vi "180122-uEye_Trigger_8bit-BM.vi"(6 "error in":errorcluster={"status"=TRUE, "code"=8, "source"="Create Folder in 170731-BM.vi<APPEND>\nC:\\Users\\FVMPE\\Desktop\\tmp\\BM"}, 8 "Phase":u16=1, 9 "Save Path":path=path "C:/Users/olfactory2P/Desktop/tmp/BM") -> (0 "error out":errorcluster={"status"=TRUE, "code"=50, "source"="LoadParameters.vi"} caption="error", 1 "DupFiles":bool)   [LabVIEW 2017]
doc: "SingleCapture_8bit nimmt ein Bilder von der Kamera auf und zeigt dieses an."
uses:
  <vilib>/vision/Image Controls.llb/IMAQ Image.ctl
  <vilib>/Analysis/_algsub.llb/Real Vector Norm.vi
  <vilib>/Analysis/Matrix/Numeric/Conversions/Array To Matrix - RA.vi
  Global_InitEndSync.vi
  <vilib>/Utility/file.llb/Write To Spreadsheet File (string).vi
  <vilib>/Analysis/Matrix/NI_Matrix.lvlib
  <vilib>/vision/NI_Vision_Development_Module.lvlib
  <vilib>/Analysis/NI_AALPro.lvlib
panel:
  in  "Settings":T1={"Objects"=1, "Threshold"=250, "Reject Border"=FALSE, "Fill Holes"=FALSE, "Min Object Size"=TRUE, "Min Size"=20, "Max Object Size"=FALSE, "Max Size"=100, "Show Search Area"=FALSE, "Show Center"=FALSE, "Show Bounding Box"=FALSE} {"Objects" items=["Bright Objects", "Dark Objects"]; "Threshold" min=1 max=999999999 step=1; "Max Size" min=1 max=999999999 step=1; "Min Size" min=1 max=999999999 step=1}
  in  "Threshold Limits":cluster{"Lower value":u8, "Upper value":u8}={"Lower value"=0, "Upper value"=66} {"Upper value" step=1 scale=0.0..255.0; "Lower value" step=1 scale=0.0..255.0}
  out "REC & Tracking State":string
  out "appended path":path
  in  "ROI to track":T2={"Left"=191, "Top"=183, "Right"=220, "Bottom"=212, "Rotation"=0.0} {"Rotation" format="%.2f"; "Left" scale=0.0..1024.0; "Right" scale=0.0..1024.0}
  out "Tracking":T3(plugin-control)
  in  "Shape Adapted Mean Shift ?":bool
  in  "Mean Shift Options in":T4={"Number of Histogram Bins"=10, "Blending Parameter (%)"=20.0, "Max Scale Change (%)"=0.0, "Max Rotation Change  (0-180 degree)"=70.0, "Max Shape Change (%)"=20.0, "Maximum Iterations"=15}
  out "Video":u8[][](graph)
  in  "Online Parameter Setting?":bool
  in  "Exposure":bool
  in  "Frame rate":u8(slide)=20 min=1 max=51 step=1 scale=1.0..50.17813236991319
  in  "Gamma":i32(slide) min=0 max=1000 step=100 scale=0.0..1000.0
  in  "Gamma":bool
  in  "Blacklevel Offset":i32(slide)=255 min=0 max=255 scale=0.0..255.0
  in  "Exposure Time":dbl(slide)=66.62091228070176 min=0.008982456140350877 max=66.62091228070176 step=0.05487719298245614 scale=0.008982456140350877..66.62091228070176 scale format="%#.3g"
  in  "Edge Filter Enable / Disable":bool
  in  "Edge Filter":i32(ring)=2 items=["High"=1, "Low"=2]
  in  "Blacklevel Compensation":bool
  in  "Hotpixel correction":bool
  in  "Master Gain":i32(slide)=100 min=0 max=100 scale=0.0..100.0
  in  "Autogain":bool
  in  "Load Parameter?":bool=TRUE
  in  "Parameter Path":path=path "C:/Users/olfactory2P/Documents/3mBM/CamParams/CamParam-180205-BM.ini"
  out "FPS":dbl=157.75358889414736
  in  "Camera ID":u32
  out "Get Trigger Mode":u16(ring)=4097 items=["Off"=0, "Hi-Low"=4097, "Low-Hi"=4098, "Software"=4104]
  in  "Trigger Mode":i32(ring)=4097 items=["IS_SET_TRIGGER_OFF"=0, "IS_SET_TRIGGER_HI_LO"=4097, "IS_SET_TRIGGER_LO_HI"=4098, "IS_SET_TRIGGER_SOFTWARE"=4104, "IS_GET_EXTERNALTRIGGER"=32768, "IS_GET_TRIGGER_STATUS"=32769]
  out "Height":i32=404
  out "Width":i32=404
  out "Bits/Pixel":i32=8
  in  "REC Stop":bool
  # "Setting"
  # "Image information"
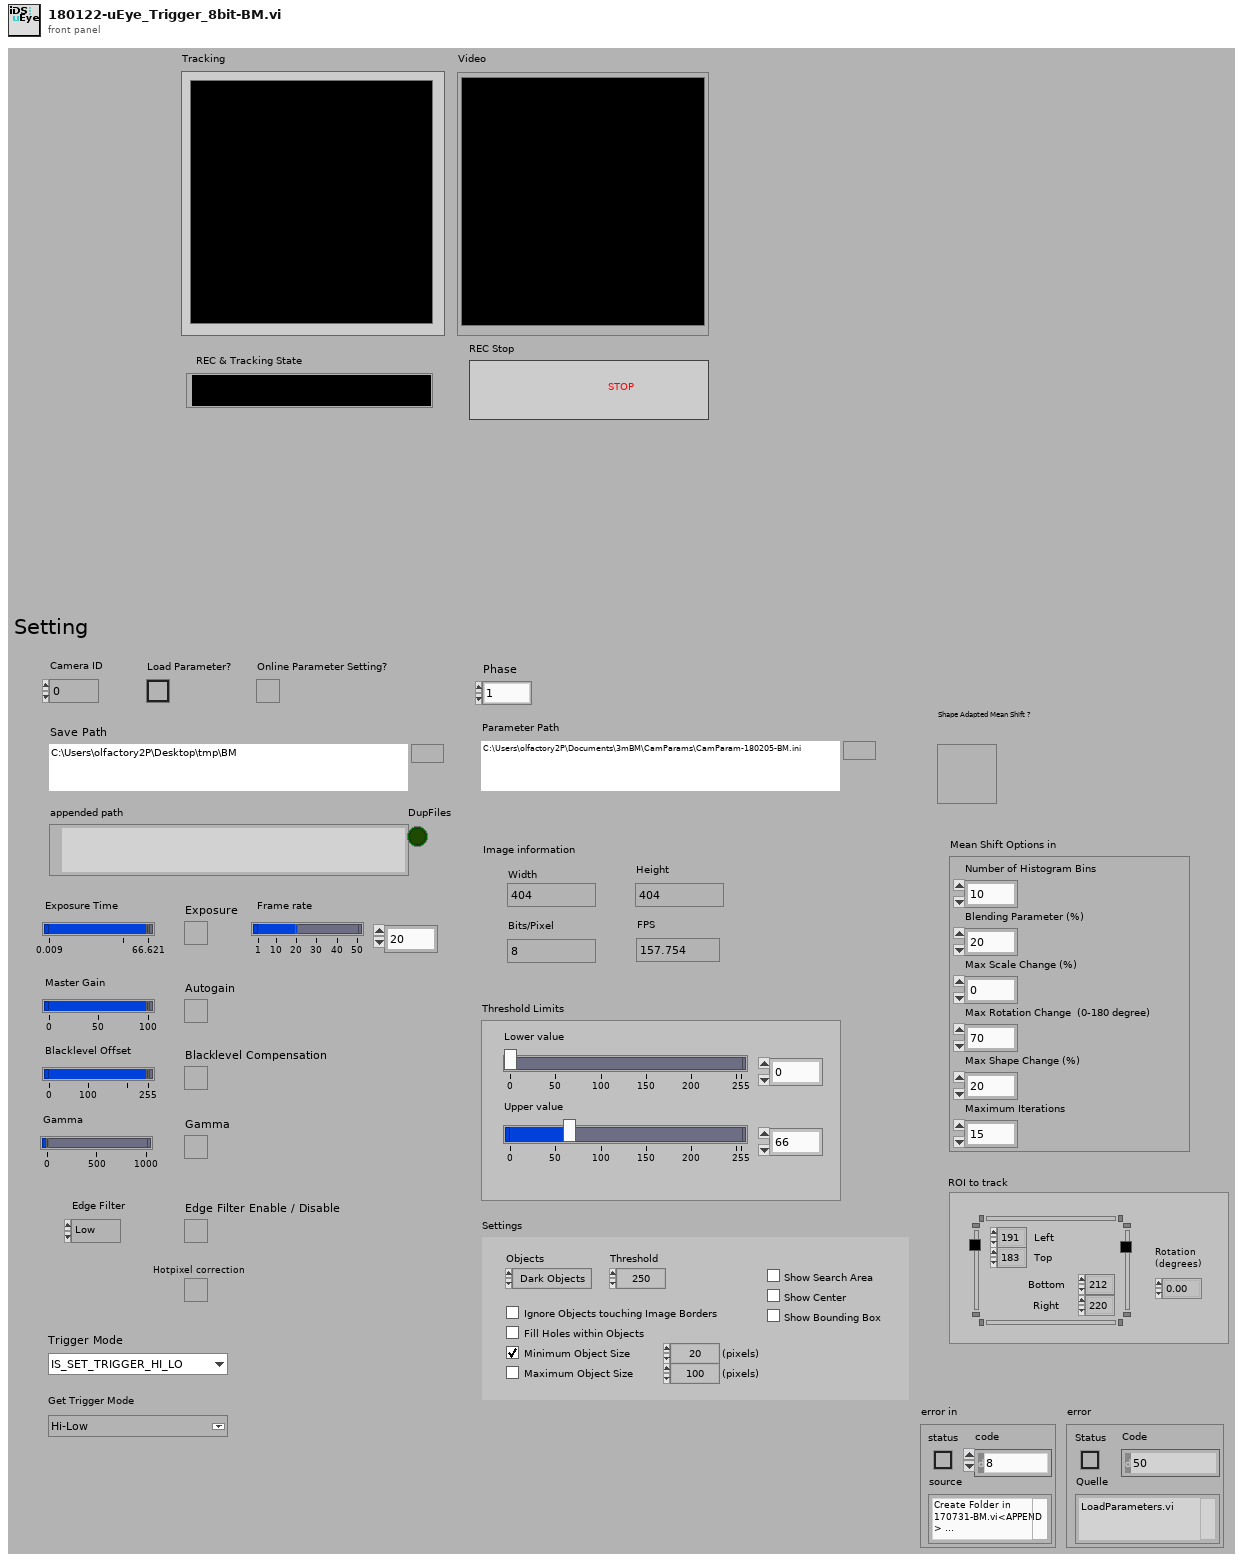
[diagram p1: front panel]
types:
  T1 = cluster{"Objects":u16, "Threshold":i32, "Reject Border":bool, "Fill Holes":bool, "Min Object Size":bool, "Min Size":i32, "Max Object Size":bool, "Max Size":i32, "Show Search Area":bool, "Show Center":bool, "Show Bounding Box":bool}
  T2 = typedef "IMAQ Rectangle" = cluster{"Left":i32, "Top":i32, "Right":i32, "Bottom":i32, "Rotation":dbl}
  T3 = typedef "IMAQ Image.ctl" = refnum<image>
  T4 = cluster{"Number of Histogram Bins":i32, "Blending Parameter (%)":dbl, "Max Scale Change (%)":dbl, "Max Rotation Change  (0-180 degree)":dbl, "Max Shape Change (%)":dbl, "Maximum Iterations":i32}
  T5 = typedef "IMAQ Object Tracking Session.ctl" = refnum<k20>
  T6 = cluster{"Number of Histogram Bins":i32, "Blending Parameter (%)":dbl, "Maximum Iterations":i32}
  T7 = typedef "IMAQ AVI2 Refnum.ctl" = refnum<k20>
  T8 = typedef "Image Type" = u32
  T9 = typedef "NI_Matrix.lvlib/RealMatrix.ctl" = dbl[][]
  T10 = cluster{"Left":i32, "Top":i32, "Right":i32, "Bottom":i32}
  T11 = typedef "ROI Descriptor" = cluster{"Global Rectangle":i32[], "Contours":cluster{"ID":enum32{"External", "Internal"}, "Type":u32, "Coordinates":i32[]}[]}
  T12 = cluster{"Label":string, "Score":i32, "Angle":dbl, "Location":cluster{"X":dbl, "Y":dbl}, "Bounding Box":cluster{"X":dbl, "Y":dbl}[], "Object Found?":bool}[]
  T13 = cluster{"Label":string, "Score":i32, "Angle":dbl, "Location":cluster{"X":dbl, "Y":dbl}, "Bounding Box":cluster{"X":dbl, "Y":dbl}[], "Object Found?":bool}
  T14 = cluster{"Object Center":cluster{"X":sgl, "Y":sgl}, "Bounding Box":cluster{"X Left":i32, "Y Top":i32, "X Right":i32, "Y Bottom":i32}, "Area":sgl, "Orientation":sgl, "Aspect Ratio":sgl, "Nb Holes":i32}[]
  T15 = cluster{"Object Center":cluster{"X":sgl, "Y":sgl}, "Bounding Box":cluster{"X Left":i32, "Y Top":i32, "X Right":i32, "Y Bottom":i32}, "Area":sgl, "Orientation":sgl, "Aspect Ratio":sgl, "Nb Holes":i32}
  T16 = cluster{"X Left":i32, "Y Top":i32, "X Right":i32, "Y Bottom":i32}
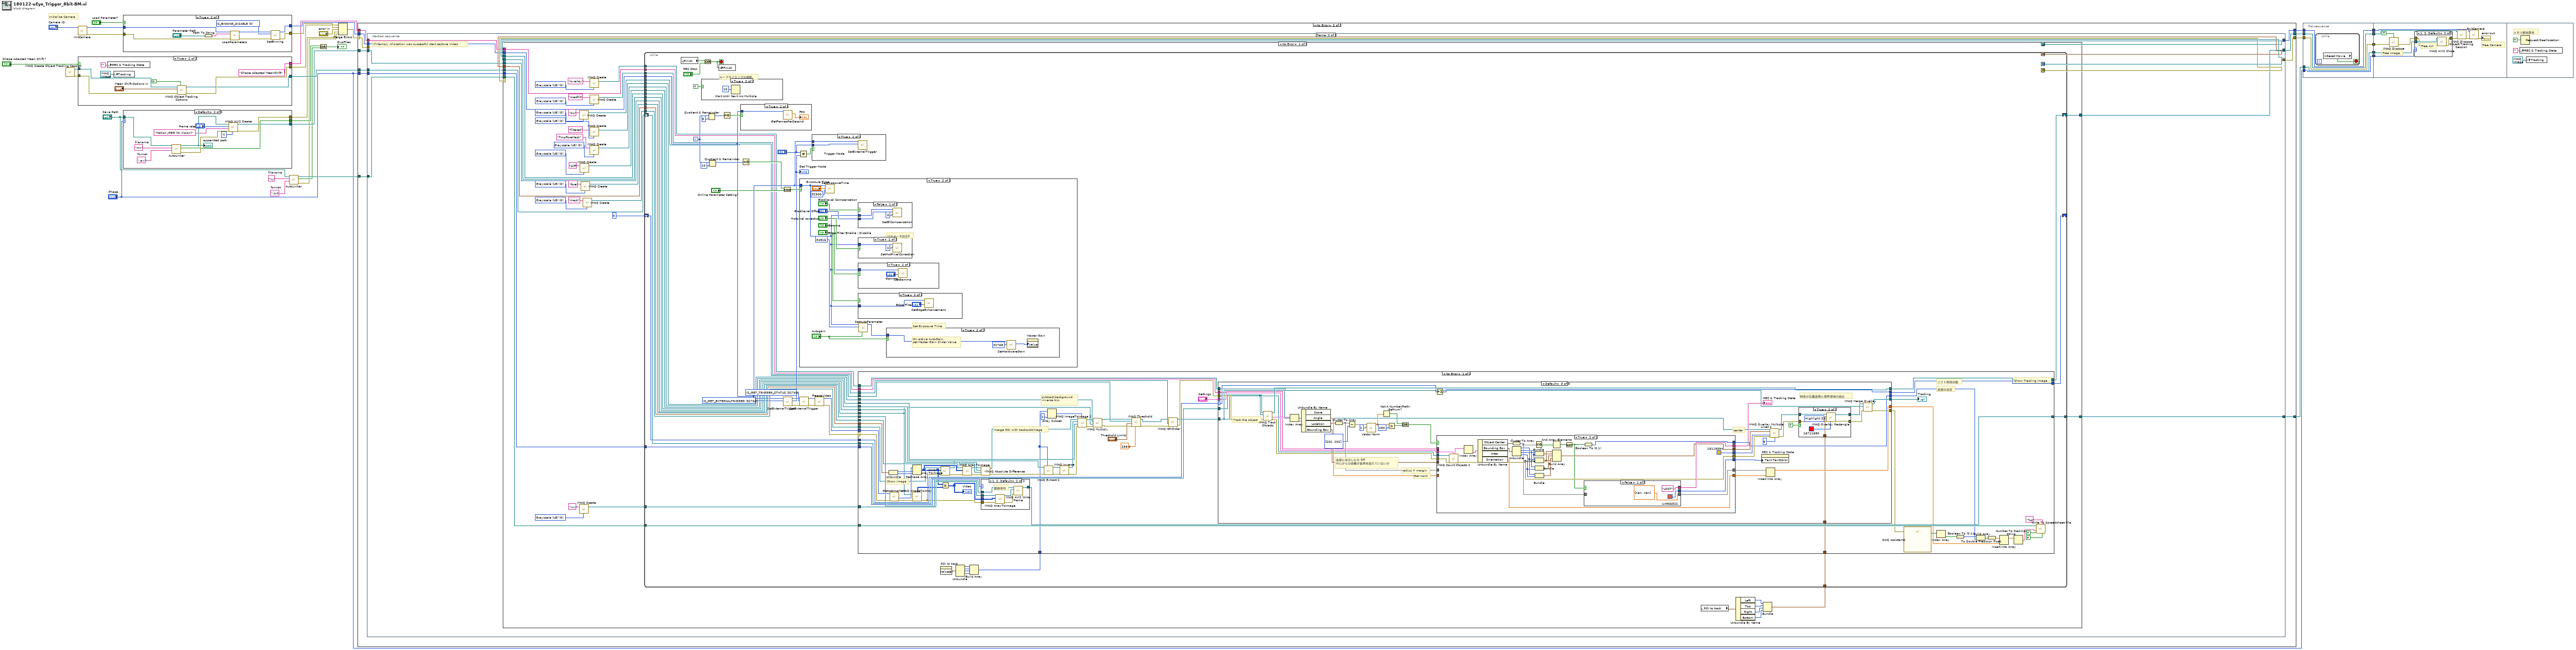
[diagram p0: block diagram]
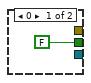
[diagram p2: hidden frame]
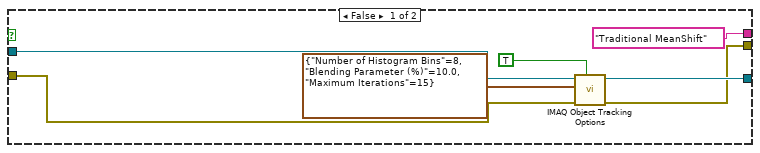
[diagram p3: hidden frame]
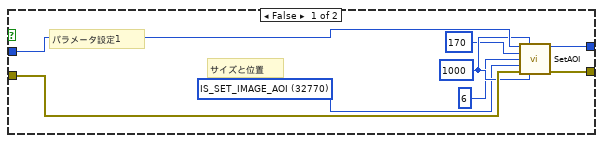
[diagram p5: hidden frame]
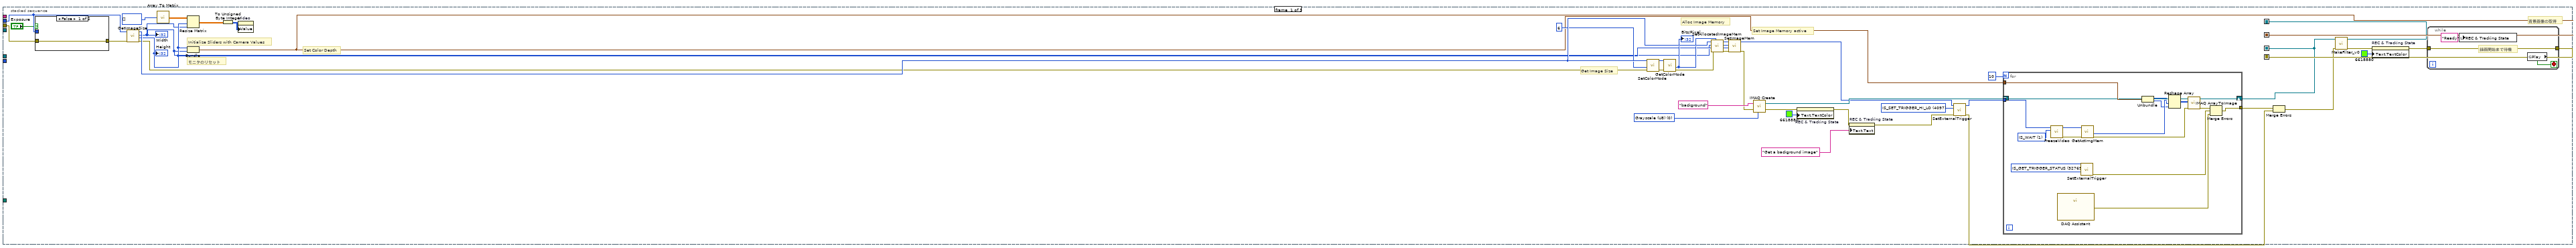
[diagram p7: hidden frame]
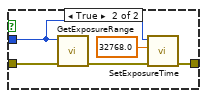
[diagram p8: hidden frame]
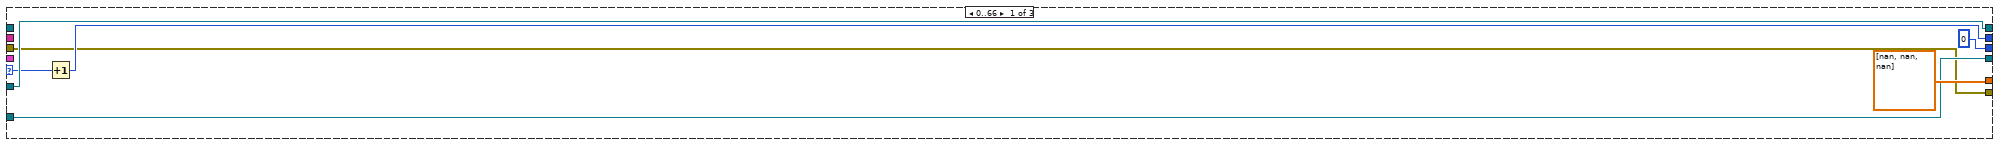
[diagram p10: hidden frame]
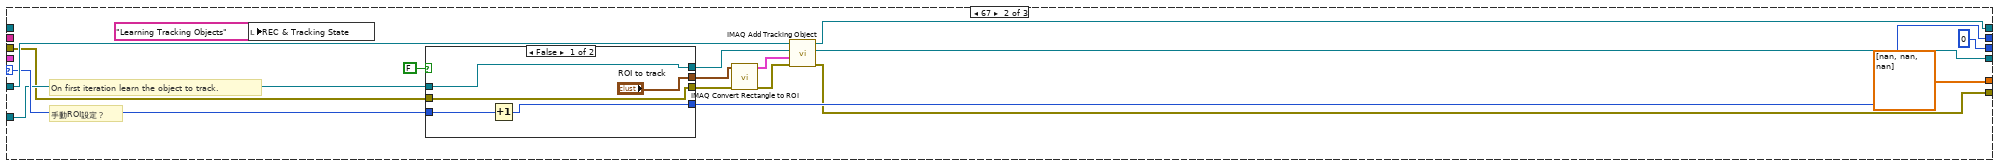
[diagram p11: hidden frame]
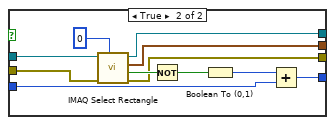
[diagram p12: hidden frame]
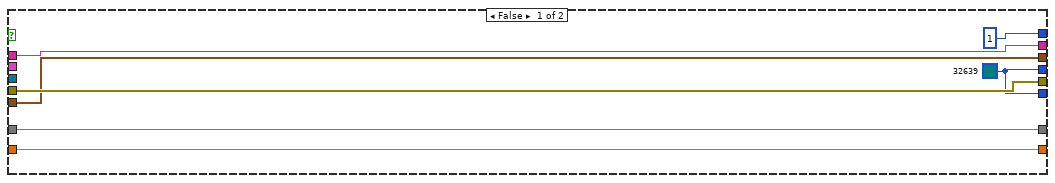
[diagram p14: hidden frame]
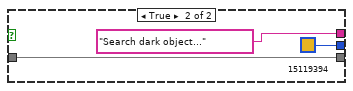
[diagram p15: hidden frame]
diagram:
  w14 = "xy"  # filename
  w13 = ".txt"  # format
  # "Initialize Camera"
  n1 = call "IMAQ Create Object Tracking Session"() -> ("error out"=w24:errorcluster, "Object Tracking Session"=w25:T5)  [unwired: 1 in, 9 out]
  n2 = call <instrlib>:"InitCamera.vi"("Camera ID"="Camera ID") -> ("error out"=w32:errorcluster, "Camera Handle Out"=w33:u32)  [unwired: 9 in]
  n3 = case shown="True" "Shape Adapted Mean Shift ?" {
    tunnel: w25 -> [w38 w50]
    tunnel: w24 -> [w37 w49]
    tunnel: [w39 w48] -> w21
    tunnel: [w40 w47] -> w20
    tunnel: ["Traditional MeanShift" "Shape Adapted MeanShift"] -> w7
    frame False {
      n4 = call-poly "IMAQ Object Tracking Options"("Get/Set (Get)"=TRUE, "error in (no error)"=w37, "Mean Shift Options in"=T6 {"Number of Histogram Bins"=8, "Blending Parameter (%)"=10.0, "Maximum Iterations"=15}, "Object Tracking Session In"=w38) -> ("error out"=w39:errorcluster, "Object Tracking Session Out"=w40:T5)  [unwired: 5 in, 1 out]
    }
    frame True {
      n5 = local write "REC & Tracking State"("") -> ()
      n6 = local write "Tracking"(T3 refnum ("Tracking")) -> ()
      n7 = call-poly "IMAQ Object Tracking Options"("Get/Set (Get)"=TRUE, "error in (no error)"=w49, "Shape Adapted Options in"="Mean Shift Options in", "Object Tracking Session In"=w50) -> ("error out"=w48:errorcluster, "Object Tracking Session Out"=w47:T5)  [unwired: 5 in, 1 out]
    }
  }
  n8 = case shown="True" "Load Parameter?" {
    tunnel: w33 -> [w58 w67]
    tunnel: [w51 w61] -> w27
    tunnel: w32 -> [w57 w66]
    tunnel: [w52 w60] -> w28
    frame False {
      w53 = 32770 items=["IS_SET_IMAGE_AOI"=32770, "IS_GET_IMAGE_AOI"=32771] ("Mode")
      w56 = 1000
      # "サイズと位置"
      # "パラメータ設定1"
      n9 = call <instrlib>:"SetAOI.vi"("Camera Handle In"=w58, "Width In"=w56, "XPos In"=170, "YPos In"=6, "Mode"=w53, "error in"=w57, "Height In"=w56) -> ("Camera Handle Out"=w51:u32, "error out"=w52:errorcluster)  [unwired: 3 in, 4 out]
    }
    frame True {
      w59 = 0 items=["IS_BINNING_DISABLE"=0, "IS_BINNING_2X_VERTICAL"=1, "IS_BINNING_2X_HORIZONTAL"=2, "IS_BINNING_4X_VERTICAL"=4, "IS_BINNING_4X_HORIZONTAL"=8, "IS_GET_BINNING"=32768, "IS_GET_SUPPORTED_BINNING"=32769] ("Mode")
      n10 = Path To String(path="Parameter Path") -> (string=w62:string)
      n11 = call <instrlib>:"LoadParameters.vi"("Camera Handle In"=w67, "Filename"=w62, "error in"=w66) -> ("Camera Handle Out"=w65:u32, "error out"=w64:errorcluster)  [unwired: 11 in]
      n12 = call <instrlib>:"SetBinning.vi"("error in"=w64, "Mode"=w59, "Camera Handle In"=w65) -> ("error out"=w60:errorcluster, "Camera Handle Out"=w61:u32)  [unwired: 6 in, 1 out]
    }
  }
  n13 = case shown="Default" "Phase" {
    tunnel: [_ w79] -> w19
    tunnel: "Save Path" -> [_ w77]
    tunnel: [_ w72] -> w15
    tunnel: [FALSE w71] -> w9
    frame 0 {
    }
    frame Default {
      w75 = "mv"  # filename
      w76 = ".avi"  # format
      n14 = call "AutoLinker.vi"("format"=w76, "filename"=w75, "Save Path"=w77) -> ("error out"=w73:errorcluster, "DupFiles"=w71:bool, "appended path"=w74:path)  [unwired: 6 in]
      "appended path" <- w74
      n15 = call "IMAQ AVI2 Create"("Quality"=-1, "error in (no error)"=w73, "Codec"="Motion JPEG (NI Vision)", "Frames Per Second"="Frame rate", "AVI Path"=w74) -> ("error out"=w72:errorcluster, "AVI Refnum"=w79:T7)  [unwired: 5 in]
    }
  }
  n16 = call "AutoLinker.vi"("format"=w13, "filename"=w14, "Save Path"="Save Path") -> ("error out"=w11:errorcluster, "DupFiles"=w10:bool, "appended path"=w16:path)  [unwired: 6 in]
  n17 = Or(x=w9, y=w10) -> (x .or. y?=→"DupFiles":bool)
  n18 = Merge Errors(w28, w21, "error in", w15, w11) -> (w30:errorcluster)
  n19 = case shown="No Error" w30 {
    selector: w30 -> [w80 w89]
    tunnel: [w81 w92] -> w29
    tunnel: w27 -> [w81 w91]
    tunnel: [w80 w90] -> w6
    tunnel: [_ w88] -> w26
    tunnel: w19 -> [_ w87]
    tunnel: w20 -> [_ w86]
    tunnel: "Phase" -> [_ w85]
    tunnel: [_ w84] -> w18
    tunnel: w16 -> [_ w83]
    tunnel: w7 -> [_ w82]
    frame Error {
    }
    frame No Error {
      n20 = stacked-sequence {
        seq-local: [w121 _ _] -> [_ w174 _]
        seq-local: [w120 _ _] -> [_ w173 w538]
        seq-local: [w100 _ _] -> [_ w168 _]
        seq-local: [w103 _ _] -> [_ w163 _]
        tunnel: w91 -> [w135 w172 w534]
        tunnel: [_ _ w530] -> w92
        tunnel: [_ _ w538] -> w90
        tunnel: w89 -> [w131 _ _]
        tunnel: [_ w171 _] -> w88
        tunnel: w87 -> [_ w170 _]
        tunnel: w86 -> [_ w167 _]
        tunnel: w85 -> [_ w169 _]
        tunnel: [_ w166 _] -> w84
        tunnel: w83 -> [_ w165 _]
        tunnel: w82 -> [_ w164 _]
        frame #0 {
          w98 = 4097 items=["IS_SET_TRIG_OFF"=0, "IS_SET_TRIG_HI_LO"=1, "IS_SET_TRIG_LO_HI"=2, "IS_SET_TRIG_SOFTWARE"=8, "IS_SET_TRIGGER_HI_LO"=4097, "IS_SET_TRIGGER_LO_HI"=4098, "IS_SET_TRIGGER_SOFTWARE"=4104, "IS_GET_EXTERNALTRIGGER"=32768, "IS_GET_TRIGGER_STATUS"=32769] ("Trigger Mode")
          w118 = T8 0 items=["Grayscale (U8)", "Grayscale (I16)", "Grayscale (SGL)", "Complex (CSG)", "RGB (U32)", "HSL (U32)", "RGB (U64)", "Grayscale (U16)"] ("Image Type")
          # "Alloc Image Memory"
          # "背景画像の取得"
          # "モニタのリセット"
          # "Initialize Sliders with Camera Values"
          # "Set Image Memory active"
          # "Set Color Depth"
          # "Get Image Size"
          n21 = case shown="False" "Exposure" {
            tunnel: w135 -> [_ w162]
            tunnel: w131 -> [w157 w160]
            tunnel: [w157 w158] -> w126
            frame False {
            }
            frame True {
              n22 = call <instrlib>:"GetExposureRange.vi"("error in"=w160, "Camera Handle In"=w162) -> ("error out"=w159:errorcluster)  [unwired: 5 in, 4 out]
              n23 = call <instrlib>:"SetExposureTime.vi"("error in"=w159, "Exposure Time"=32768.0, "Camera Handle In"=w162) -> ("error out"=w158:errorcluster)  [unwired: 6 in, 2 out]
            }
          }
          n24 = call <instrlib>:"GetImageSize.vi"("error in"=w126, "Camera Handle In"=w135) -> ("error out"=w130:errorcluster, "Height"=w123:i32, "Width"=w111:i32, "Camera Handle Out"=w136:u32)  [unwired: 6 in]
          "Width" <- w111
          "Height" <- w123
          n25 = call-poly <vilib>:"Array To Matrix.vi"("Real 1D Array"=i32[] []) -> ("Real Matrix (Column Vector)"=w125:T9)
          n26 = Resize Matrix(1:w111, 2:w123, 4:w125) -> (0:w122:T9)
          n27 = Bundle("Height"=w123, "Width"=w111) -> (w121:cluster{"Height":i32, "Width":i32})  [unwired: 1 in]
          n28 = To Unsigned Byte Integer(number=w122) -> (unsigned 8bit integer=w112:u8[][])
          n29 = property on="Video" class="IntGraph (strict)"("Value"=w112) -> ()  [unwired: 2 in, 2 out]
          n30 = call <instrlib>:"SetColorMode.vi"("error in"=w130, "Mode"=6, "Camera Handle In"=w136) -> ("error out"=w129:errorcluster, "Camera Handle Out"=w134:u32)  [unwired: 7 in]
          n31 = call <instrlib>:"GetColorMode.vi"("error in"=w129, "Camera Handle In"=w134) -> ("error out"=w128:errorcluster, "Bits/Pixel"=w132:i32)  [unwired: 6 in, 2 out]
          "Bits/Pixel" <- w132
          n32 = call <instrlib>:"SetAllocatedImageMem.vi"("BitsPixel"=w132, "error in"=w128, "Height"=w123, "Width"=w111, "Camera Handle In"=w136) -> ("error out"=w109:errorcluster, "Image Memory Out"=w110:u8[], "Memory ID Out"=w107:i32, "Camera Handle Out"=w108:u32)  [unwired: 2 in, 1 out]
          n33 = call <instrlib>:"SetImageMem.vi"("error in"=w109, "Image Memory In"=w110, "Memory ID In"=w107, "Camera Handle In"=w108) -> ("error out"=w117:errorcluster, "Camera Handle Out"=w97:u32)  [unwired: 4 in, 2 out]
          n34 = call "IMAQ Create"("Image Name"="background", "Image Type"=w118, "error in (no error)"=w117) -> ("New Image"=w106:T3, "error out"=w113:errorcluster)  [unwired: 2 in]
          n35 = property on="REC & Tracking State" class="Str"(error in=w113, "Text.TextColor"=u32 6618880 ("Color")) -> (error out=w101:errorcluster)  [unwired: 1 in, 1 out]
          n36 = property on="REC & Tracking State" class="Str"(error in=w101, "Text.Text"="Get a background image") -> (error out=w95:errorcluster)  [unwired: 1 in, 1 out]
          n37 = call <instrlib>:"SetExternalTrigger.vi"("error in"=w95, "Trigger Mode"=w98, "Camera Handle In"=w97) -> ("error out"=w94:errorcluster, "Camera Handle Out"=w96:u32)  [unwired: 6 in, 1 out]
          n38 = for {
            N: 10 -> [_]
            tunnel: w121 -> [w153]
            tunnel: [w151] -> w105
            tunnel: w96 -> [w149]
            shift-right: [w150] -> w100
            shift-left: w106 -> [w152]
            w140 = 1 items=["IS_DONT_WAIT", "IS_WAIT"] ("Wait")
            w143 = 32769 items=["IS_SET_TRIG_OFF"=0, "IS_SET_TRIG_HI_LO"=1, "IS_SET_TRIG_LO_HI"=2, "IS_SET_TRIG_SOFTWARE"=8, "IS_SET_TRIGGER_HI_LO"=4097, "IS_SET_TRIGGER_LO_HI"=4098, "IS_SET_TRIGGER_SOFTWARE"=4104, "IS_GET_EXTERNALTRIGGER"=32768, "IS_GET_TRIGGER_STATUS"=32769] ("Trigger Mode")
            n39 = call <instrlib>:"FreezeVideo.vi"("Wait"=w140, "Camera Handle In"=w149) -> ("error out"=w141:errorcluster, "Camera Handle Out"=w142:u32)  [unwired: 8 in]
            n40 = call "DAQ Assistant"() -> ("error out"=w137:errorcluster)  [unwired: 18 in, 1 out]
            n41 = call <instrlib>:"SetExternalTrigger.vi"("Trigger Mode"=w143) -> ("error out"=w138:errorcluster)  [unwired: 8 in, 2 out]
            n42 = call <instrlib>:"GetActImgMem.vi"("error in"=w141, "Camera Handle In"=w142) -> ("error out"=w144:errorcluster, "Image Memory Out"=w148:u8[])  [unwired: 6 in, 2 out]
            n43 = Unbundle(w153) -> ("Height"=w147:i32, "Width"=w146:i32)
            n44 = Reshape Array(w148, w147, w146) -> (w145:u8[][])
            n45 = call "IMAQ ArrayToImage"("error in (no error)"=w144, "Image Pixels (U8)"=w145, "Image"=w152) -> ("error out"=w139:errorcluster, "Image Out"=w150:T3)  [unwired: 7 in]
            n46 = Merge Errors(w139, w138, w137) -> (w151:errorcluster)
          }
          n47 = Merge Errors(w105, w94) -> (w99:errorcluster)
          n48 = call "MakeFilter_v0.vi"("error in (no error)"=w99, "Image"=w100) -> ("error out"=w104:errorcluster, "Image Out"=w103:T3)  [unwired: 8 in]
          n49 = property on="REC & Tracking State" class="Str"(error in=w104, "Text.TextColor"=u32 6618880 ("Color")) -> (error out=w115:errorcluster)  [unwired: 1 in, 1 out]
          n50 = while {
            tunnel: w115 -> [w155]
            tunnel: [w155] -> w120
            stop <- w156 stop-if-true
            # "録画開始まで待機"
            n51 = local write "REC & Tracking State"("Ready") -> ()
            n52 = global read "Global_InitEndSync.vi" "Play"() -> (w156:bool)
          }
        }
        frame #1 {
          # "If Memory Allocation was successful start capture Video"
          n53 = case shown="No Error" w173 {
            tunnel: w172 -> [w218 _]
            tunnel: w174 -> [w219 _]
            tunnel: [w216 _] -> w171
            tunnel: w170 -> [w217 _]
            tunnel: w167 -> [w210 _]
            tunnel: w169 -> [w212 _]
            tunnel: w168 -> [w211 _]
            tunnel: [w208 _] -> w166
            tunnel: w165 -> [w204 _]
            tunnel: w164 -> [w188 _]
            tunnel: w163 -> [w184 _]
            frame No Error {
              w183 = T8 0 items=["Grayscale (U8)", "Grayscale (I16)", "Grayscale (SGL)", "Complex (CSG)", "RGB (U32)", "HSL (U32)", "RGB (U64)", "Grayscale (U16)"] ("Image Type")
              w187 = T8 0 items=["Grayscale (U8)", "Grayscale (I16)", "Grayscale (SGL)", "Complex (CSG)", "RGB (U32)", "HSL (U32)", "RGB (U64)", "Grayscale (U16)"] ("Image Type")
              w191 = T8 0 items=["Grayscale (U8)", "Grayscale (I16)", "Grayscale (SGL)", "Complex (CSG)", "RGB (U32)", "HSL (U32)", "RGB (U64)", "Grayscale (U16)"] ("Image Type")
              w194 = T8 0 items=["Grayscale (U8)", "Grayscale (I16)", "Grayscale (SGL)", "Complex (CSG)", "RGB (U32)", "HSL (U32)", "RGB (U64)", "Grayscale (U16)"] ("Image Type")
              w198 = T8 0 items=["Grayscale (U8)", "Grayscale (I16)", "Grayscale (SGL)", "Complex (CSG)", "RGB (U32)", "HSL (U32)", "RGB (U64)", "Grayscale (U16)"] ("Image Type")
              w199 = T8 0 items=["Grayscale (U8)", "Grayscale (I16)", "Grayscale (SGL)", "Complex (CSG)", "RGB (U32)", "HSL (U32)", "RGB (U64)", "Grayscale (U16)"] ("Image Type")
              w202 = T8 0 items=["Grayscale (U8)", "Grayscale (I16)", "Grayscale (SGL)", "Complex (CSG)", "RGB (U32)", "HSL (U32)", "RGB (U64)", "Grayscale (U16)"] ("Image Type")
              w207 = T8 0 items=["Grayscale (U8)", "Grayscale (I16)", "Grayscale (SGL)", "Complex (CSG)", "RGB (U32)", "HSL (U32)", "RGB (U64)", "Grayscale (U16)"] ("Image Type")
              w209 = T8 0 items=["Grayscale (U8)", "Grayscale (I16)", "Grayscale (SGL)", "Complex (CSG)", "RGB (U32)", "HSL (U32)", "RGB (U64)", "Grayscale (U16)"] ("Image Type")
              n54 = call "IMAQ Create"("Image Name"="bw", "Image Type"=w199) -> ("New Image"=w197:T3)  [unwired: 3 in, 1 out]
              n55 = call "IMAQ Create"("Image Name"="inv", "Image Type"=w198) -> ("New Image"=w196:T3)  [unwired: 3 in, 1 out]
              n56 = call "IMAQ Create"("Image Name"="diff", "Image Type"=w191) -> ("New Image"=w189:T3)  [unwired: 3 in, 1 out]
              n57 = call "IMAQ Create"("Image Name"="fore", "Image Type"=w209) -> ("New Image"=w213:T3)  [unwired: 3 in, 1 out]
              n58 = call "IMAQ Create"("Image Name"="mask", "Image Type"=w207) -> ("New Image"=w205:T3)  [unwired: 3 in, 1 out]
              n59 = call "IMAQ Create"("Image Name"="overlay", "Image Type"=w194) -> ("New Image"=w193:T3)  [unwired: 3 in, 1 out]
              n60 = call "IMAQ Create"("Image Name"="medfilt", "Image Type"=w187) -> ("New Image"=w185:T3)  [unwired: 3 in, 1 out]
              n61 = call "IMAQ Create"("Image Name"="filtered", "Image Type"=w183) -> ("New Image"=w181:T3)  [unwired: 3 in, 1 out]
              n62 = call "IMAQ Create"("Image Name"="TmpForeMask", "Image Type"=w202) -> ("New Image"=w201:T3)  [unwired: 3 in, 1 out]
              n63 = local read "ROI to track"() -> (w176:T2)
              n64 = Unbundle By Name(w176) -> ("Left"=w177:i32, "Top"=w178:i32, "Right"=w179:i32, "Bottom"=w180:i32)
              n65 = Bundle("Left"=w177, "Top"=w178, "Right"=w179, "Bottom"=w180) -> (w175:T10)  [unwired: 1 in]
              n66 = while {
                tunnel: w219 -> [w264]
                tunnel: w218 -> [w261]
                tunnel: [w266] -> w216
                tunnel: w217 -> [w263]
                shift-right: [w249] -> _
                shift-left: 0 -> [w246]
                tunnel: w213 -> [w248]
                tunnel: w212 -> [w245]
                tunnel: w211 -> [w243]
                shift-right: [w242] -> w208
                shift-left: w210 -> [w241]
                tunnel: w205 -> [w240]
                tunnel: w204 -> [w239]
                tunnel: w201 -> [w238]
                tunnel: w197 -> [w235]
                tunnel: w196 -> [w234]
                tunnel: w193 -> [w233]
                tunnel: w189 -> [w232]
                tunnel: w188 -> [w231]
                tunnel: w185 -> [w230]
                tunnel: w184 -> [w228]
                tunnel: w181 -> [w227]
                tunnel: w175 -> [w226]
                i -> [w253]
                stop <- w229 stop-if-true
                w247 = 32769 items=["IS_SET_TRIG_OFF"=0, "IS_SET_TRIG_HI_LO"=1, "IS_SET_TRIG_LO_HI"=2, "IS_SET_TRIG_SOFTWARE"=8, "IS_SET_TRIGGER_HI_LO"=4097, "IS_SET_TRIGGER_LO_HI"=4098, "IS_SET_TRIGGER_SOFTWARE"=4104, "IS_GET_EXTERNALTRIGGER"=32768, "IS_GET_TRIGGER_STATUS"=32769] ("Trigger Mode")
                w262 = 32768 items=["IS_SET_TRIG_OFF"=0, "IS_SET_TRIG_HI_LO"=1, "IS_SET_TRIG_LO_HI"=2, "IS_SET_TRIG_SOFTWARE"=8, "IS_SET_TRIGGER_HI_LO"=4097, "IS_SET_TRIGGER_LO_HI"=4098, "IS_SET_TRIGGER_SOFTWARE"=4104, "IS_GET_EXTERNALTRIGGER"=32768, "IS_GET_TRIGGER_STATUS"=32769] ("Trigger Mode")
                # "ループタイミングの調節"
                n67 = global read "Global_InitEndSync.vi" "Finish"() -> (w255:bool)
                n68 = case shown="True" TRUE {
                  frame False {
                  }
                  frame True {
                    n69 = Wait Until Next ms Multiple(millisecond multiple=u32 10) -> ()  [unwired: 1 out]
                  }
                }
                n70 = Or(x=w255, y="REC Stop") -> (x .or. y?=w229:bool)
                n71 = Quotient & Remainder(x=w253, y=5) -> (x-y*floor(x/y)=w272:i32)  [unwired: 1 out]
                n72 = Quotient & Remainder(x=w253, y=10) -> (x-y*floor(x/y)=w269:i32)  [unwired: 1 out]
                n73 = global write "Global_InitEndSync.vi" "Finish"(w229) -> ()
                n74 = Equal To 0?(x=w272) -> (x = 0?=w271:bool)
                n75 = case shown="True" w271 {
                  tunnel: w261 -> [_ w521]
                  frame False {
                  }
                  frame True {
                    n76 = call <instrlib>:"GetFramesPerSecond.vi"("Camera Handle In"=w521) -> ("FPS"=→"FPS":dbl)  [unwired: 8 in, 2 out]
                  }
                }
                n77 = Equal To 0?(x=w269) -> (x = 0?=w260:bool)
                n78 = And(x=w260, y="Online Parameter Setting?") -> (x .and. y?=w265:bool)
                n79 = call <instrlib>:"SetExternalTrigger.vi"("Trigger Mode"=w262, "Camera Handle In"=w261) -> ("error out"=w250:errorcluster, "Status"=w244:i32, "Camera Handle Out"=w251:u32)  [unwired: 7 in]
                "Get Trigger Mode" <- w244
                n80 = Not Equal?(x="Trigger Mode", y=w244) -> (x != y?=w257:bool)
                n81 = case shown="True" w265 {
                  tunnel: w261 -> [_ w488]
                  frame False {
                  }
                  frame True {
                    # "パラメータ設定2"
                    # "Set Exposure Time"
                    n82 = call <instrlib>:"SetExposureTime.vi"("Mode"=u16 32900, "Exposure Time"="Exposure Time", "Camera Handle In"=w488) -> ()  [unwired: 6 in, 3 out]
                    n83 = case shown="False" "Blacklevel Compensation" {
                      tunnel: w488 -> [w507 w510]
                      tunnel: "Blacklevel Offset" -> [w505 w508]
                      frame False {
                        n84 = call <instrlib>:"SetBlCompensation.vi"("Mode"=0, "offset"=w505, "Camera Handle In"=w507) -> ()  [unwired: 6 in, 3 out]
                      }
                      frame True {
                        n85 = call <instrlib>:"SetBlCompensation.vi"("Mode"=1, "offset"=w508, "Camera Handle In"=w510) -> ()  [unwired: 6 in, 3 out]
                      }
                    }
                    n86 = case shown="True" "Hotpixel correction" {
                      tunnel: w488 -> [w512 w514]
                      frame False {
                        n87 = call <instrlib>:"SetHotPixelCorrection.vi"("Mode"=0, "Camera Handle In"=w512) -> ()  [unwired: 7 in, 3 out]
                      }
                      frame True {
                        n88 = call <instrlib>:"SetHotPixelCorrection.vi"("Mode"=2, "Camera Handle In"=w514) -> ()  [unwired: 7 in, 3 out]
                      }
                    }
                    n89 = case shown="True" "Gamma" {
                      tunnel: w488 -> [_ w500]
                      frame False {
                      }
                      frame True {
                        n90 = call <instrlib>:"SetGamma.vi"("Gamma"="Gamma", "Camera Handle In"=w500) -> ()  [unwired: 8 in, 2 out]
                      }
                    }
                    n91 = case shown="True" "Edge Filter Enable / Disable" {
                      tunnel: w488 -> [w501 w504]
                      frame False {
                        n92 = call <instrlib>:"SetEdgeEnhancement.vi"("Mode"=0, "Camera Handle In"=w501) -> ()  [unwired: 8 in, 2 out]
                      }
                      frame True {
                        n93 = call <instrlib>:"SetEdgeEnhancement.vi"("Mode"="Edge Filter", "Camera Handle In"=w504) -> ()  [unwired: 8 in, 2 out]
                      }
                    }
                    n94 = call <instrlib>:"SetAutoParameter.vi"("enable"="Autogain", "Param"=34816, "Camera Handle In"=w488) -> ("Camera Handle Out"=w497:u32)  [unwired: 6 in, 2 out]
                    n95 = case shown="True" "Autogain" {
                      tunnel: w497 -> [w515 w518]
                      frame False {
                        # "Set Master Gain"
                        n96 = call <instrlib>:"SetHardwareGain.vi"("Master Gain"="Master Gain", "Camera Handle In"=w515) -> ()  [unwired: 7 in, 3 out]
                      }
                      frame True {
                        # "On active AutoGain,\nset Master Gain Slider Value"
                        n97 = call <instrlib>:"SetHardwareGain.vi"("Mode"=32768, "Camera Handle In"=w518) -> ("Value"=w519:i32)  [unwired: 7 in, 2 out]
                        n98 = property on="Master Gain" class="Slide (strict)"("Value"=w519) -> ()  [unwired: 2 in, 2 out]
                      }
                    }
                  }
                }
                n99 = call <instrlib>:"SetExternalTrigger.vi"("error in"=w250, "Trigger Mode"=w247, "Camera Handle In"=w251) -> ("error out"=w237:errorcluster, "Camera Handle Out"=w252:u32)  [unwired: 6 in, 1 out]
                n100 = case shown="True" w257 {
                  tunnel: w261 -> [_ w487]
                  tunnel: "Trigger Mode" -> [_ w486]
                  frame False {
                  }
                  frame True {
                    n101 = call <instrlib>:"SetExternalTrigger.vi"("Trigger Mode"=w486, "Camera Handle In"=w487) -> ()  [unwired: 7 in, 3 out]
                  }
                }
                n102 = call <instrlib>:"FreezeVideo.vi"("error in"=w237, "Camera Handle In"=w252) -> ("error out"=w236:errorcluster, "Camera Handle Out"=w254:u32)  [unwired: 8 in]
                n103 = property on="ROI to track" class="Clust (strict)"() -> ("Value"=w225:T2)  [unwired: 2 in, 2 out]
                n104 = Unbundle(w225) -> ("Left"=w224:i32, "Top"=w223:i32, "Right"=w222:i32, "Bottom"=w221:i32)  [unwired: 1 out]
                n105 = Build Array(w224, w223, w222, w221) -> (w220:i32[])
                n106 = case shown="No Error" w236 {
                  selector: w236 -> [w335 _]
                  tunnel: [w342 w484] -> w266
                  tunnel: w264 -> [w341 _]
                  tunnel: w263 -> [w340 w484]
                  tunnel: w254 -> [w339 _]
                  tunnel: w241 -> [w334 w482]
                  tunnel: [w330 w483] -> w249
                  tunnel: w246 -> [w331 w483]
                  tunnel: w248 -> [w315 _]
                  tunnel: w245 -> [w333 _]
                  tunnel: w243 -> [w310 _]
                  tunnel: [w332 w482] -> w242
                  tunnel: w240 -> [w314 _]
                  tunnel: w239 -> [w327 _]
                  tunnel: w238 -> [w308 _]
                  tunnel: w235 -> [w280 _]
                  tunnel: w234 -> [w293 _]
                  tunnel: w233 -> [w305 _]
                  tunnel: w232 -> [w304 _]
                  tunnel: w231 -> [w302 _]
                  tunnel: w230 -> [w299 _]
                  tunnel: w228 -> [w287 _]
                  tunnel: w227 -> [w298 _]
                  tunnel: w226 -> [w275 _]
                  tunnel: w220 -> [w273 _]
                  frame No Error {
                    # "subtract background,\ninverse b/w"
                    # "merge ROI with backsubtImage"
                    # "追尾の成否"
                    # "Show Tracking Image"
                    # "リフト昇降状態"
                    # "Show Image"
                    n107 = Unbundle(w341) -> ("Height"=w338:i32, "Width"=w337:i32)
                    n108 = call <instrlib>:"GetActImgMem.vi"("error in"=w335, "Camera Handle In"=w339) -> ("error out"=w284:errorcluster, "Image Memory Out"=w336:u8[])  [unwired: 6 in, 2 out]
                    n109 = Reshape Array(w336, w338, w337) -> (w286:u8[][])
                    n110 = call "IMAQ ImageToArray"("error in (no error)"=w284, "Image"=w287) -> ("error out"=w283:errorcluster, "Image Pixels (U8)"=w288:u8[][])  [unwired: 2 in, 3 out]
                    n111 = call "IMAQ ArrayToImage"("error in (no error)"=w283, "Image Pixels (U8)"=w286, "Image"=w314) -> ("error out"=w306:errorcluster, "Image Out"=w309:T3)  [unwired: 7 in]
                    n112 = Multiply(x=w286, y=w288) -> (x*y=w285:u8[][])
                    "Video" <- w285
                    n113 = call "IMAQ ArrayToImage"("error in (no error)"=w306, "Image Pixels (U8)"=w286, "Image"=w315) -> ("error out"=w307:errorcluster, "Image Out"=w311:T3)  [unwired: 7 in]
                    n114 = call "IMAQ Absolute Difference"("Image Src A"=w311, "Image Dst"=w304, "Image Src B"=w310, "error in (no error)"=w307) -> ("Image Dst Out"=w295:T3, "error out"=w294:errorcluster)  [unwired: 3 in]
                    n115 = case shown="1, 2, Default" w333 {
                      tunnel: [w343 w350] -> w342
                      tunnel: w340 -> [w343 w349]
                      tunnel: w293 -> [_ w348]
                      tunnel: w283 -> [_ w347]
                      tunnel: w285 -> [_ w346]
                      frame 0 {
                      }
                      frame 1, 2, Default {
                        # "動画保存"
                        n116 = call "IMAQ ArrayToImage"("error in (no error)"=w347, "Image Pixels (U8)"=w346, "Image"=w348) -> ("error out"=w345:errorcluster, "Image Out"=w344:T3)  [unwired: 7 in]
                        n117 = call "IMAQ AVI2 Write Frame"("error in (no error)"=w345, "Image"=w344, "AVI Refnum"=w349) -> ("AVI Refnum (duplicate)"=w350:T7)  [unwired: 6 in, 2 out]
                      }
                    }
                    n118 = call "IMAQ Extract 2"("Optional Rectangle"=w273, "error in (no error)"=w294, "Image Src"=w309) -> ("error out"=w291:errorcluster, "Image Dst Out"=w292:T3)  [unwired: 7 in]
                    n119 = Array Subset(array=w273, length=2) -> (w312:i32[])  [unwired: 1 in]
                    n120 = call "IMAQ Inverse"("error in (no error)"=w291, "Image Src"=w292) -> ("error out"=w289:errorcluster, "Image Dst Out"=w290:T3)  [unwired: 8 in]
                    n121 = call "IMAQ ImageToImage 2"("Offset Left/Top"=w312, "error in (no error)"=w289, "Image Dst"=w308, "Image Src (Small)"=w290, "Image Src (Large)"=w295) -> ("error out"=w296:errorcluster, "Image Dst Out"=w297:T3)  [unwired: 5 in]
                    n122 = call "IMAQ Multiply"("Image Src A"=w297, "Image Dst"=w298, "Image Src B"=w287, "error in (no error)"=w296) -> ("Image Dst Out"=w282:T3, "error out"=w281:errorcluster)  [unwired: 3 in]
                    n123 = call "IMAQ Threshold"("Replace Value"=255.0, "error in (no error)"=w281, "Range"="Threshold Limits", "Image Dst"=w280, "Image Src"=w282) -> ("error out"=w278:errorcluster, "Image Dst Out"=w279:T3)  [unwired: 5 in]
                    n124 = call "IMAQ NthOrder"("Image Src"=w279, "Image Dst"=w299, "error in (no error)"=w278) -> ("Image Dst Out"=w300:T3, "error out"=w301:errorcluster)  [unwired: 4 in]
                    n125 = case shown="Default" w331 {
                      selector: w331 -> [w356 w369 w427]
                      tunnel: [w357 w373 w432] -> w332
                      tunnel: w334 -> [w357 w374 w431]
                      tunnel: [w352 w359 w413] -> w316
                      tunnel: [w355 w366 w404] -> w330
                      tunnel: [dbl[] [nan, nan, nan] ("Location") dbl[] [nan, nan, nan] ("Location") w408] -> w318
                      tunnel: [0 0 w410] -> w320
                      tunnel: w301 -> [w351 w360 w397]
                      tunnel: w300 -> [w352 w361 w396]
                      tunnel: w305 -> [_ _ w395]
                      tunnel: "Settings" -> [_ _ w394]
                      tunnel: w302 -> [_ _ w393]
                      tunnel: w275 -> [_ _ w392]
                      tunnel: [w351 w358 w391] -> w274
                      frame 0..66 {
                        n126 = Increment(x=w356) -> (x+1=w355:i32)
                      }
                      frame 67 {
                        # "手動ROI設定？"
                        # "On first iteration learn the object to track."
                        n127 = local write "REC & Tracking State"("Learning Tracking Objects") -> ()
                        n128 = case shown="False" FALSE {
                          tunnel: w361 -> [w378 w389]
                          tunnel: w369 -> [w379 w385]
                          tunnel: [w377 w384] -> w366
                          tunnel: [w378 w383] -> w368
                          tunnel: ["ROI to track" w382] -> w367
                          tunnel: w360 -> [w376 w381]
                          tunnel: [w376 w380] -> w362
                          frame False {
                            n129 = Increment(x=w379) -> (x+1=w377:i32)
                          }
                          frame True {
                            n130 = call "IMAQ Select Rectangle"("Window Number (0...15)"=0, "error in (no error)"=w381, "Image In"=w389) -> ("error out"=w380:errorcluster, "Cancelled"=w388:bool, "Rectangle"=w382:T2, "Image Out (duplicate)"=w383:T3)  [unwired: 5 in]
                            n131 = Not(x=w388) -> (.not. x?=w387:bool)
                            n132 = Boolean To (0,1)(Boolean=w387) -> (0, 1=w386:i16)
                            n133 = Add(x=w386, y=w385) -> (x+y=w384:i32)
                          }
                        }
                        n134 = call "IMAQ Convert Rectangle to ROI"("error in (no error)"=w362, "Rectangle"=w367) -> ("error out"=w372:errorcluster, "ROI Descriptor"=w371:T11)  [unwired: 7 in]
                        n135 = call "IMAQ Add Tracking Object"("error in (no error)"=w372, "ROI Descriptor"=w371, "Image"=w368, "Object Tracking Session In"=w374) -> ("error out"=w358:errorcluster, "Image (duplicate)"=w359:T3, "Object Tracking Session Out"=w373:T5)  [unwired: 1 in, 4 out]
                      }
                      frame Default {
                        # "追尾に成功したか OR \n中心からの距離が基準を超えていないか"
                        # "Get norm"
                        # "center"
                        # "radius + margin"
                        # "物体の位置座標と境界領域の抽出"
                        # "Track the object"
                        n136 = call "IMAQ Track Objects"("error in (no error)"=w397, "Image"=w396, "Object Tracking Session In"=w431) -> ("error out"=w428:errorcluster, "Objects (pixel)"=w418:T12, "Object Tracking Session Out"=w432:T5)  [unwired: 1 in, 5 out]
                        n137 = Index Array(array=w418) -> (element=w430:T13)  [unwired: 1 in]
                        n138 = Unbundle By Name(w430) -> ("Angle"=w406:dbl, "Location"=w429:cluster{"X":dbl, "Y":dbl}, "Bounding Box"=w414:cluster{"X":dbl, "Y":dbl}[])  [unwired: 1 out]
                        n139 = Cluster To Array(cluster=w429) -> (array=w412:dbl[])
                        n140 = Subtract(x=w412, y=i32[] [202, 202]) -> (x-y=w424:dbl[])
                        n141 = call-poly <vilib>:"Vector Norm.vi"("norm type"=1, "Input Vector"=w424) -> ("norm"=w423:dbl)  [unwired: 8 in, 1 out]
                        n142 = Not A Number/Path/Refnum?(number/path/refnum=w423) -> (NaN/Path/Refnum?=w421:bool)
                        n143 = Greater?(x=w423, y=250) -> (0:w420:bool)
                        n144 = Or(x=w421, y=w420) -> (x .or. y?=w411:bool)
                        n145 = Increment(x=w427) -> (x+1=w404:i32)
                        n146 = case shown="True" w411 {
                          tunnel: w428 -> [w448 w470]
                          tunnel: [w448 w469] -> w417
                          tunnel: w396 -> [_ w471]
                          tunnel: [w444 u32 15119394 ("Color")] -> w416
                          tunnel: [w446 w449] -> w419
                          tunnel: [w447 w453] -> w415
                          tunnel: w414 -> [w447 _]
                          tunnel: w412 -> [w446 _]
                          tunnel: [1 w475] -> w410
                          tunnel: [w442 w474] -> w403
                          tunnel: [w444 w473] -> w405
                          tunnel: [w443 w464] -> w407
                          tunnel: w406 -> [w443 _]
                          tunnel: w394 -> [_ w462]
                          tunnel: w393 -> [w442 _]
                          frame False {
                            w444 = u32 32639 ("Color")
                          }
                          frame True {
                            n147 = call "IMAQ Count Objects 2"("Settings"=w462, "error in (no error)"=w470, "Image"=w471) -> ("error out"=w469:errorcluster, "Objects"=w468:T14)  [unwired: 4 in, 3 out]
                            n148 = Index Array(array=w468) -> (element=w467:T15)  [unwired: 1 in]
                            n149 = Unbundle By Name(w467) -> ("Object Center"=w465:cluster{"X":sgl, "Y":sgl}, "Bounding Box"=w466:T16, "Orientation"=w464:sgl)  [unwired: 1 out]
                            n150 = Cluster To Array(cluster=w465) -> (array=w450:sgl[])
                            n151 = Unbundle(w466) -> ("X Left"=w461:i32, "Y Top"=w458:i32, "X Right"=w460:i32, "Y Bottom"=w459:i32)
                            n152 = Equal To 0?(x=w450) -> (x = 0?=w463:bool[])
                            n153 = Bundle("X Right"=w460, "Y Top"=w458) -> (w456:cluster{"X Right":i32, "Y Top":i32})  [unwired: 1 in]
                            n154 = Bundle("X Left"=w461, "Y Top"=w458) -> (w457:cluster{"X Left":i32, "Y Top":i32})  [unwired: 1 in]
                            n155 = Bundle("X Right"=w460, "Y Bottom"=w459) -> (w455:cluster{"X Right":i32, "Y Bottom":i32})  [unwired: 1 in]
                            n156 = Bundle("X Left"=w461, "Y Bottom"=w459) -> (w454:cluster{"X Left":i32, "Y Bottom":i32})  [unwired: 1 in]
                            n157 = And Array Elements(Boolean array=w463) -> (logical AND=w452:bool)
                            n158 = Build Array(w457, w456, w455, w454, w457) -> (w453:cluster{"X Left":i32, "Y Top":i32}[])
                            n159 = Not(x=w452) -> (.not. x?=w451:bool)
                            n160 = Boolean To (0,1)(Boolean=w451) -> (0, 1=w475:i16)
                            n161 = case shown="False" w451 {
                              tunnel: ["LOST" "Search dark object..."] -> w474
                              tunnel: [u32 14966322 ("Color") u32 15119394 ("Color")] -> w473
                              tunnel: w450 -> [_ w479]
                              tunnel: [dbl[] [nan, nan] w479] -> w449
                              frame False {
                              }
                              frame True {
                              }
                            }
                          }
                        }
                        "REC & Tracking State" <- w403
                        n162 = property on="REC & Tracking State" class="Str"("Text.TextColor"=w405) -> ()  [unwired: 2 in, 2 out]
                        n163 = Insert Into Array(array=w419, new element=w407) -> (w408:dbl[])  [unwired: 1 in]
                        n164 = call "IMAQ Overlay Multiple Lines 2"("Image"=w396, "Line End Points"=w415, "Color"=w416, "error in (no error)"=w417, "Width"=5) -> ("Image Out"=w401:T3, "error out"=w400:errorcluster)  [unwired: 9 in]
                        n165 = case shown="True" TRUE {
                          tunnel: [w434 w436] -> w402
                          tunnel: w401 -> [w434 w441]
                          tunnel: w400 -> [w433 w438]
                          tunnel: [w433 w437] -> w399
                          tunnel: w392 -> [_ w440]
                          frame False {
                          }
                          frame True {
                            w435 = u32 2 items=["Frame", "Fill", "Highlight"] ("Drawing Mode (Frame)")
                            n166 = call "IMAQ Overlay Rectangle"("Color"=u32 16711680, "error in (no error)"=w438, "Drawing Mode (Frame)"=w435, "Rectangle"=w440, "Image"=w441) -> ("error out"=w437:errorcluster, "Image Out"=w436:T3)  [unwired: 5 in]
                          }
                        }
                        n167 = call "IMAQ Merge Overlay"("error in (no error)"=w399, "Image Dst"=w395, "Image Src"=w402) -> ("error out"=w391:errorcluster, "Image Dst Out"=w413:T3)  [unwired: 7 in]
                      }
                    }
                    "Tracking" <- w316
                    n168 = call "DAQ Assistant2"("error in"=w274) -> ("data"=w324:bool[])  [unwired: 16 in, 2 out]
                    n169 = Index Array(array=w324) -> (element=w323:bool)  [unwired: 1 in]
                    n170 = Boolean To (0,1)(Boolean=w323) -> (0, 1=w321:i16)
                    n171 = Build Array(w321, w320) -> (w319:i32[])
                    n172 = To Double Precision Float(number=w319) -> (double precision float=w317:dbl[])
                    n173 = Insert Into Array(array=w317, new element=w318) -> (w322:dbl[])  [unwired: 1 in]
                    n174 = Number To Decimal String(number=w322) -> (decimal integer string=w325:string[])  [unwired: 1 in]
                    n175 = call-poly <vilib>:"Write To Spreadsheet File.vi"("transpose? (no:F)"=FALSE, "format (%s)"="%s", "append to file? (new file:F)"=TRUE, "1D data"=w325, "file path (dialog if empty)"=w327) -> ()  [unwired: 3 in, 1 out]
                  }
                  frame Error {
                  }
                }
              }
            }
            frame Error {
              (unwired) ""
            }
          }
        }
        frame #2 {
          # "モニタのリセット"
          n176 = call-poly <vilib>:"Array To Matrix.vi"("Real 1D Array"=i32[] []) -> ("Real Matrix (Column Vector)"=w537:T9)
          n177 = call <instrlib>:"GetImageSize.vi"("Camera Handle In"=w534) -> ("error out"=w526:errorcluster, "Height"=w532:i32, "Width"=w533:i32, "Camera Handle Out"=w527:u32)  [unwired: 7 in]
          n178 = Resize Matrix(1:w533, 2:w532, 4:w537) -> (0:w535:T9)
          n179 = call <instrlib>:"GetActImgMem.vi"("error in"=w526, "Camera Handle In"=w527) -> ("error out"=w522:errorcluster, "Image Memory Out"=w523:u8[], "Memory Number"=w524:i32, "Camera Handle Out"=w525:u32)  [unwired: 6 in]
          n180 = To Unsigned Byte Integer(number=w535) -> (unsigned 8bit integer=w531:u8[][])
          n181 = call <instrlib>:"FreeImageMem.vi"("error in"=w522, "Image Memory"=w523, "Memory ID"=w524, "Camera Handle In"=w525) -> ("error out"=w528:errorcluster, "Camera Handle Out"=w529:u32)  [unwired: 6 in]
          n182 = local write "Video"(w531) -> ()
          n183 = call <instrlib>:"StopLiveVideo.vi"("error in"=w528, "Camera Handle In"=w529) -> ("Camera Handle Out"=w530:u32)  [unwired: 8 in, 1 out]
        }
      }
    }
  }
  n184 = flat-sequence {
    tunnel: w18 -> [w539]
    tunnel: "Phase" -> [w540]
    tunnel: w26 -> [w541]
    tunnel: w29 -> [w542]
    tunnel: w6 -> [w543]
    tunnel: [w543] -> w5
    tunnel: [w542] -> w4
    tunnel: [w541] -> w3
    tunnel: [w540] -> w2
    tunnel: [w539] -> w1
    tunnel: w5 -> [w547]
    tunnel: w4 -> [w552]
    tunnel: w3 -> [w553]
    tunnel: w2 -> [w551]
    tunnel: w1 -> [w548]
    frame #0 {
      n185 = while {
        stop <- w544 stop-if-true
        n186 = global read "Global_InitEndSync.vi" "Reset Movie"() -> (w544:bool)
      }
    }
    frame #1 {
      # "Free Image"
      # "Free Camera"
      n187 = call "IMAQ Dispose"("All Images? (No)"=TRUE, "error in (no error)"=w547) -> ("error out"=w546:errorcluster)  [unwired: 4 in]
      n188 = case shown="1, 2, Default" w551 {
        tunnel: w553 -> [_ w558]
        tunnel: w546 -> [w555 w557]
        tunnel: [w555 w556] -> w550
        frame 0 {
        }
        frame 1, 2, Default {
          # "Free AVI"
          n189 = call "IMAQ AVI2 Close"("error in (no error)"=w557, "AVI Refnum"=w558) -> ("error out"=w556:errorcluster)  [unwired: 9 in]
        }
      }
      n190 = call "IMAQ Dispose Object Tracking Session"("error in (no error)"=w550, "Object Tracking Session"=w548) -> ("error out"=w549:errorcluster)  [unwired: 9 in]
      n191 = call <instrlib>:"ExitCamera.vi"("error in"=w549, "Camera Handle In"=w552) -> ("error out"=→"error out":errorcluster)  [unwired: 9 in]
    }
    frame #2 {
      # "メモリ解放要求"
      n192 = local write "REC & Tracking State"("") -> ()
      n193 = Request Deallocation(TRUE ("メモリ開放要求？")) -> ()
      n194 = local write "Tracking"(T3 refnum ("Tracking")) -> ()
    }
  }
